vi "run_auto EAE0_test .vi"(8 "error in (no error)":errorcluster, 9 "user event out":T1, 10 "modbusData":refnum<notifier>, 11 "Cluster":T2) -> (0 "error out":errorcluster)   [LabVIEW 2019]
uses:
  core_dataRefCluster.ctl
  core_dataRef.ctl
  core_dataCluster.ctl
  instrument/instr_dataCluster.ctl
  gui/test_result_user_event.ctl
  core_autoMonitorDataCluster.ctl
  limits/report_mode.ctl
  <vilib>/Platform/TimedLoop/XDataNode/timing_clust.ctl
  <vilib>/Platform/TimedLoop/XDataNode/nitl_modes.ctl
  <vilib>/Platform/TimedLoop/XDataNode/wakeup.ctl
  <vilib>/Platform/TimedLoop/XDataNode/XDataNode.xnode
  <vilib>/Platform/TimedLoop/XDataNode/XDNodeRunTimeDep.lvlib
  instrument/Instrument.lvclass
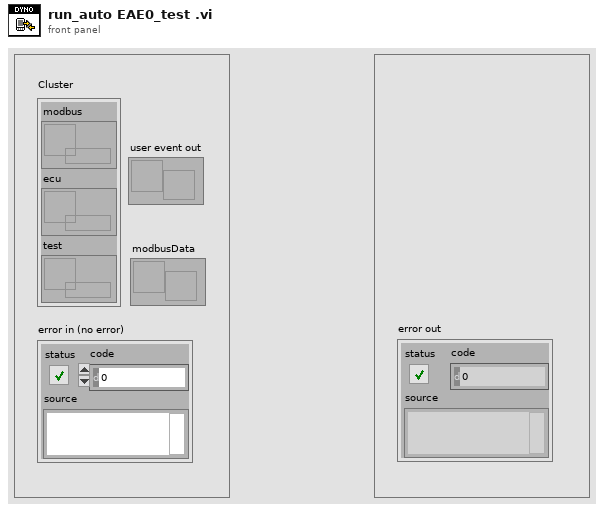
[diagram p1: front panel]
types:
  T1 = typedef "test_result_user_event.ctl" = refnum<user-event>
  T2 = typedef "core_dataRefCluster.ctl" = cluster{"modbus":T3, "ecu":T3, "test":T3}
  T3 = typedef "core_dataRef.ctl" = refnum<queue>
  T4 = typedef "report_mode.ctl" = enum16{"Initialize", "Save", "Close"}
  T5 = typedef "core_dataCluster.ctl" = cluster{"cmd":string, "data":variant}
  T6 = typedef "XDNodeRunTimeDep.lvlib/timing_clust.ctl" = cluster{"Expected End [f-1]":u64, "Actual End [f-1]":u64, "Finished Late? [f-1]":bool, "Expected End [i-1]":u64, "Actual End [i-1]":u64, "Finished Late? [i-1]":bool, "Expected Start [i]":u64, "Actual Start [i]":u64, "Expected Start [f]":u64, "Actual Start [f]":u64, "Source Name":string, "Structure Name":string, "Period":i64, "Deadline":i64, "Offset":i64, "Start":i64, "Priority":i32, "Timeout":i32, "Mode":T7, "Wakeup Reason":T8, "Error":errorcluster, "Source Type":string, "Secondary Source Type":string, "Global End Time":u64, "Global Start Time":u64, "Frame Duration":u64, "Iteration Duration":u64, "Assigned CPU":i32, "I/O Scan Engine Mode":u32}
  T7 = typedef "XDNodeRunTimeDep.lvlib/nitl_modes.ctl" = enum32{"No Change", "Process missed periods, maintain original phase", "Discard missed periods, maintain original phase", "Process missed periods, ignore original phase", "Discard missed periods, ignore original phase"}
  T8 = typedef "XDNodeRunTimeDep.lvlib/wakeup.ctl" = enum32{"Normal", "Aborted", "Asynchronous wakeup", "Timing source error", "Timed loop error", "Timeout"}
  T9 = typedef "limits_limitList.ctl" = cluster{"sec":i32, "spec":T10}
  T10 = typedef "limits_specs.ctl" = cluster{"torque":dbl, "lower_speed":dbl, "upper_speed":dbl, "input_power":dbl, "output_power":dbl, "efficiency":dbl}
  T11 = typedef "core_autoMonitorDataCluster.ctl" = cluster{"torque":dbl, "speed":dbl, "input power":dbl, "output power":dbl, "efficiency":dbl, "DC_power":dbl, "status":bool, "torque1":bool, "rpm1":bool, "Efficiency1":bool}
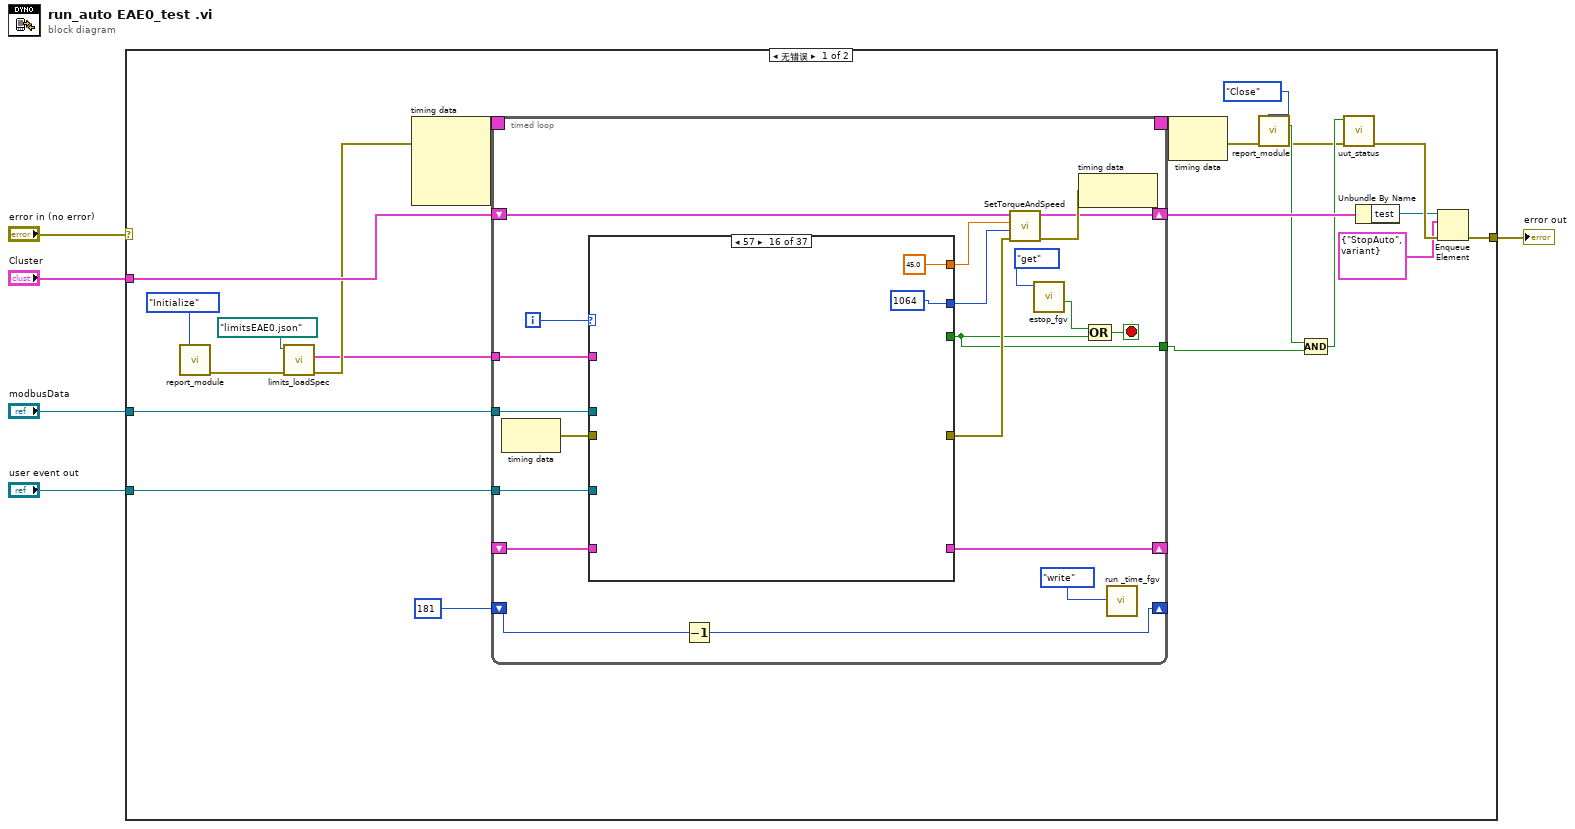
[diagram p0: block diagram]
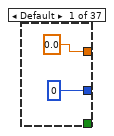
[diagram p2: hidden frame]
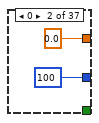
[diagram p3: hidden frame]
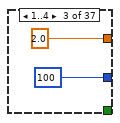
[diagram p4: hidden frame]
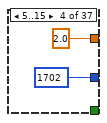
[diagram p5: hidden frame]
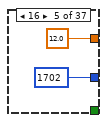
[diagram p6: hidden frame]
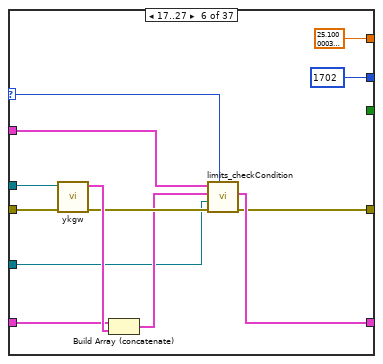
[diagram p7: hidden frame]
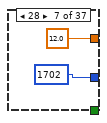
[diagram p8: hidden frame]
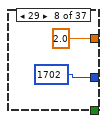
[diagram p9: hidden frame]
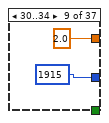
[diagram p10: hidden frame]
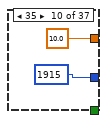
[diagram p11: hidden frame]
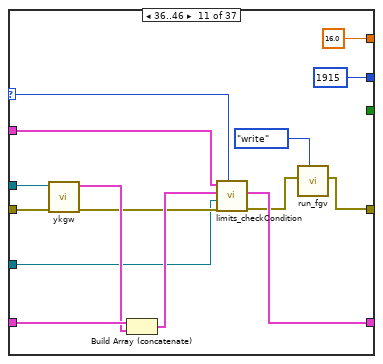
[diagram p12: hidden frame]
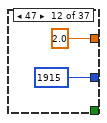
[diagram p13: hidden frame]
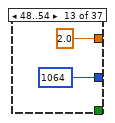
[diagram p14: hidden frame]
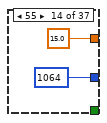
[diagram p15: hidden frame]
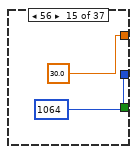
[diagram p16: hidden frame]
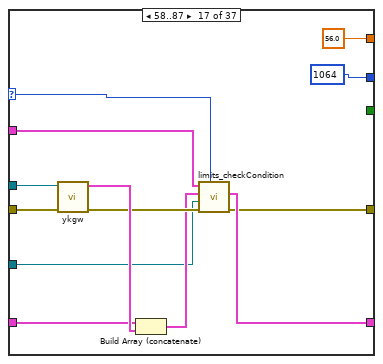
[diagram p17: hidden frame]
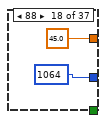
[diagram p18: hidden frame]
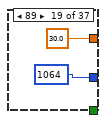
[diagram p19: hidden frame]
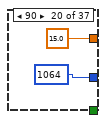
[diagram p20: hidden frame]
diagram:
  n1 = case shown="无错误" "error in (no error)" {
    selector: "error in (no error)" -> [_ w201]
    tunnel: "Cluster" -> [w20 _]
    tunnel: [w24 w201] -> w4
    tunnel: "modbusData" -> [w19 _]
    tunnel: "user event out" -> [w13 _]
    frame No Error {
      n2 = call "report_module.vi"("mode"=report_mode."Initialize") -> ("error out"=w12:errorcluster)  [unwired: 9 in, 5 out]
      n3 = call "limits_loadSpec.vi"("error in (no error)"=w12, "limits file"=path "limitsEAE0.json") -> ("error out"=w18:errorcluster, "test limits"=w17:T9[])  [unwired: 8 in]
      n4 = node-c288(w18) -> (w22:T6)  [unwired: 3 in]
      n5 = timed-loop {
        timing: w22 -> [_]
        timing-out: [_] -> w21
        shift-right: [w44] -> w26
        shift-left: w20 -> [w47]
        tunnel: w19 -> [w40]
        shift-right: [w37] -> _
        shift-left: _ -> [w36]
        tunnel: w17 -> [w35]
        tunnel: w13 -> [w33]
        shift-right: [w29] -> _
        shift-left: 181 -> [w30]
        tunnel: [w31] -> w14
        i -> [w28]
        stop <- w41 stop-if-true
        n6 = node-c288() -> (w39:errorcluster)  [unwired: 1 in]
        n7 = case shown="57" w28 {
          selector: w28 -> [_ _ _ _ _ w61 _ _ _ _ w89 _ _ _ _ _ w104 _ _ _ _ _ w129 _ w144 _ _ _ _ _ w172 _ _ _ _ _ _]
          tunnel: [sgl 0.0 ("Torque") sgl 0.0 ("Torque") sgl 2.0 ("Torque") sgl 2.0 ("Torque") sgl 12.0 ("Torque") sgl 25.1 ("Torque") sgl 12.0 ("Torque") sgl 2.0 ("Torque") sgl 2.0 ("Torque") sgl 10.0 ("Torque") sgl 16.0 ("Torque") sgl 2.0 ("Torque") sgl 2.0 ("Torque") sgl 15.0 ("Torque") sgl 30.0 ("Torque") sgl 45.0 ("Torque") sgl 56.0 ("Torque") sgl 45.0 ("Torque") sgl 30.0 ("Torque") sgl 15.0 ("Torque") sgl 2.0 ("Torque") sgl 2.0 ("Torque") sgl 12.5 ("Torque") sgl 20.0 ("Torque") sgl 20.0 ("Torque") sgl 10.0 ("Torque") sgl 2.0 ("Torque") sgl 2.0 ("Torque") sgl 15.0 ("Torque") sgl 30.0 ("Torque") sgl 42.0 ("Torque") sgl 30.0 ("Torque") sgl 15.0 ("Torque") sgl 2.0 ("Torque") sgl 2.0 ("Torque") sgl 0.0 ("Torque") sgl 0.0 ("Torque")] -> w42
          tunnel: [0 ("Speed") 100 ("Speed") 100 ("Speed") 1702 ("Speed") 1702 ("Speed") 1702 ("Speed") 1702 ("Speed") 1702 ("Speed") 1915 ("Speed") 1915 ("Speed") 1915 ("Speed") 1915 ("Speed") 1064 ("Speed") 1064 ("Speed") 1064 ("Speed") 1064 ("Speed") 1064 ("Speed") 1064 ("Speed") 1064 ("Speed") 1064 ("Speed") 1064 ("Speed") 3404 ("Speed") 3404 ("Speed") 3404 ("Speed") 3404 ("Speed") 3404 ("Speed") 2404 ("Speed") 1702 ("Speed") 1702 ("Speed") 1702 ("Speed") 1702 ("Speed") 1702 ("Speed") 1702 ("Speed") 1702 ("Speed") 100 ("Speed") 100 ("Speed") 0 ("Speed")] -> w45
          tunnel: [_ _ _ _ _ _ _ _ _ _ _ _ _ _ _ _ _ _ _ _ _ _ _ _ _ _ _ _ _ _ _ _ _ _ _ _ TRUE] -> w31
          tunnel: w40 -> [_ _ _ _ _ w68 _ _ _ _ w91 _ _ _ _ _ w113 _ _ _ _ _ w132 _ w146 _ _ _ _ _ w170 _ _ _ _ _ _]
          tunnel: w39 -> [_ _ _ _ _ w66 _ _ _ _ w90 _ _ _ _ _ w112 _ _ _ _ _ w128 _ w145 _ _ _ _ _ w169 _ _ _ _ _ _]
          tunnel: [_ _ _ _ _ w59 _ _ _ _ w81 _ _ _ _ _ w106 _ _ _ _ _ w130 _ w142 _ _ _ _ _ w166 _ _ _ _ _ _] -> w38
          tunnel: [_ _ _ _ _ w60 _ _ _ _ w84 _ _ _ _ _ w108 _ _ _ _ _ w131 _ w147 _ _ _ _ _ w167 _ _ _ _ _ _] -> w37
          tunnel: w36 -> [_ _ _ _ _ w65 _ _ _ _ w87 _ _ _ _ _ w110 _ _ _ _ _ w136 _ w151 _ _ _ _ _ w168 _ _ _ _ _ _]
          tunnel: w35 -> [_ _ _ _ _ w62 _ _ _ _ w88 _ _ _ _ _ w107 _ _ _ _ _ w133 _ w148 _ _ _ _ _ w171 _ _ _ _ _ _]
          tunnel: w33 -> [_ _ _ _ _ w58 _ _ _ _ w79 _ _ _ _ _ w105 _ _ _ _ _ w127 _ w143 _ _ _ _ _ w165 _ _ _ _ _ _]
          frame Default {
          }
          frame 0 {
          }
          frame 1..4 {
          }
          frame 5..15 {
          }
          frame 16 {
          }
          frame 17..27 {
            n8 = call "ykgw.vi"("error in (no error)"=w66, "modbusData"=w68) -> ("error out"=w64:errorcluster, "Cluster"=w67:T11)  [unwired: 8 in]
            n9 = Build Array (concatenate)(w65, w67) -> (w63:T11[])
            n10 = call "limits_checkCondition.vi"("Sec"=w61, "error in (no error)"=w64, "user event out"=w58, "Data in"=w63, "test limits"=w62) -> ("error out"=w59:errorcluster, "Data out"=w60:T11[])  [unwired: 5 in]
          }
          frame 28 {
          }
          frame 29 {
          }
          frame 30..34 {
          }
          frame 35 {
          }
          frame 36..46 {
            n11 = call "ykgw.vi"("error in (no error)"=w90, "modbusData"=w91) -> ("error out"=w83:errorcluster, "Cluster"=w86:T11)  [unwired: 8 in]
            n12 = Build Array (concatenate)(w87, w86) -> (w85:T11[])
            n13 = call "limits_checkCondition.vi"("Sec"=w89, "error in (no error)"=w83, "user event out"=w79, "Data in"=w85, "test limits"=w88) -> ("error out"=w82:errorcluster, "Data out"=w84:T11[])  [unwired: 5 in]
            n14 = call "run_fgv.vi"("mode"=enum16{"read", "write"}."write", "error in (no error)"=w82) -> ("error out"=w81:errorcluster)  [unwired: 7 in, 2 out]
          }
          frame 47 {
          }
          frame 48..54 {
          }
          frame 55 {
          }
          frame 56 {
          }
          frame 57 {
          }
          frame 58..87 {
            n15 = call "ykgw.vi"("error in (no error)"=w112, "modbusData"=w113) -> ("error out"=w111:errorcluster, "Cluster"=w114:T11)  [unwired: 8 in]
            n16 = Build Array (concatenate)(w110, w114) -> (w109:T11[])
            n17 = call "limits_checkCondition.vi"("Sec"=w104, "error in (no error)"=w111, "user event out"=w105, "Data in"=w109, "test limits"=w107) -> ("error out"=w106:errorcluster, "Data out"=w108:T11[])  [unwired: 5 in]
          }
          frame 88 {
          }
          frame 89 {
          }
          frame 90 {
          }
          frame 91 {
          }
          frame 92..112 {
          }
          frame 113..123 {
            n18 = call "ykgw.vi"("error in (no error)"=w128, "modbusData"=w132) -> ("error out"=w137:errorcluster, "Cluster"=w135:T11)  [unwired: 8 in]
            n19 = Build Array (concatenate)(w136, w135) -> (w134:T11[])
            n20 = call "limits_checkCondition.vi"("Sec"=w129, "error in (no error)"=w137, "user event out"=w127, "Data in"=w134, "test limits"=w133) -> ("error out"=w130:errorcluster, "Data out"=w131:T11[])  [unwired: 5 in]
            n21 = call "run_fgv.vi"() -> ()  [unwired: 9 in, 3 out]
          }
          frame 124 {
          }
          frame 125..134 {
            n22 = call "ykgw.vi"("error in (no error)"=w145, "modbusData"=w146) -> ("error out"=w152:errorcluster, "Cluster"=w150:T11)  [unwired: 8 in]
            n23 = Build Array (concatenate)(w151, w150) -> (w149:T11[])
            n24 = call "limits_checkCondition.vi"("Sec"=w144, "error in (no error)"=w152, "user event out"=w143, "Data in"=w149, "test limits"=w148) -> ("error out"=w142:errorcluster, "Data out"=w147:T11[])  [unwired: 5 in]
          }
          frame 135 {
          }
          frame 136 {
          }
          frame 137..147 {
          }
          frame 148 {
          }
          frame 149 {
          }
          frame 150..165 {
            n25 = call "ykgw.vi"("error in (no error)"=w169, "modbusData"=w170) -> ("error out"=w174:errorcluster, "Cluster"=w175:T11)  [unwired: 8 in]
            n26 = Build Array (concatenate)(w168, w175) -> (w173:T11[])
            n27 = call "limits_checkCondition.vi"("Sec"=w172, "error in (no error)"=w174, "user event out"=w165, "Data in"=w173, "test limits"=w171) -> ("error out"=w166:errorcluster, "Data out"=w167:T11[])  [unwired: 5 in]
          }
          frame 166 {
          }
          frame 167 {
          }
          frame 168 {
          }
          frame 169..178 {
          }
          frame 179 {
          }
          frame 180 {
          }
        }
        n28 = Decrement(x=w30) -> (x-1=w29:i32)
        n29 = call "SetTorqueAndSpeed.vi"("error in (no error)"=w38, "Speed"=w45, "Torque"=w42, "Cluster in"=w47) -> ("error out"=w46:errorcluster, "Cluster out"=w44:T2)  [unwired: 6 in]
        n30 = call "estop_fgv.vi"("Enum"=enum16{"set", "get"}."get") -> ("indicator"=w34:bool)  [unwired: 9 in, 1 out]
        n31 = node-c288(w46) -> ()  [unwired: 1 out]
        n32 = Compound Arithmetic op=OR ("复合运算")(w34, w31) -> (w41:bool)
        n33 = call "run _time_fgv .vi"("mode"=enum16{"read", "write"}."write") -> ()  [unwired: 2 in, 2 out]
      }
      n34 = node-c288(w21) -> (w10:errorcluster)
      n35 = call "report_module.vi"("mode"=report_mode."Close", "error in (no error)"=w10) -> ("Passed"=w9:bool, "error out"=w8:errorcluster)  [unwired: 8 in, 4 out]
      n36 = Compound Arithmetic op=AND(w9, w14) -> (w15:bool)
      n37 = call "uut_status.vi"("error in (no error)"=w8, "status"=w15) -> ("error out"=w27:errorcluster)  [unwired: 9 in]
      n38 = Unbundle By Name(w26) -> ("test"=w25:T3)
      n39 = Enqueue Element(queue=w25, element=T5 {"cmd"="StopAuto", "data"=variant}, error in (no error)=w27) -> (error out=w24:errorcluster)  [unwired: 1 in, 2 out]
    }
    frame Error {
    }
  }
  "error out" <- w4
